vi "Cleanup.vi"(8 "error in (no error)":errorcluster, 11 "HAL Editor in":refnum<class "HAL Editor.lvclass">) -> (0 "error out":errorcluster)   [LabVIEW 2012, in "HAL Config.lvlib" / "HAL Editor.lvclass"]
uses:
  HAL Editor.lvclass
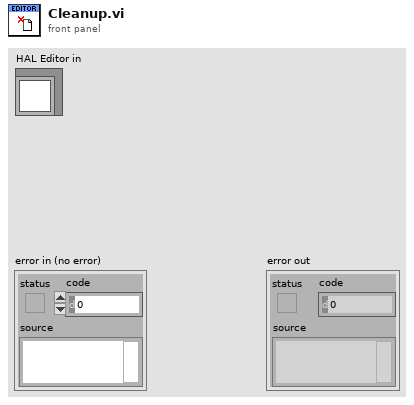
[diagram p1: front panel]
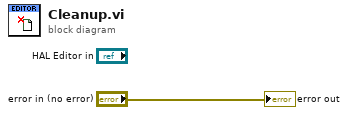
[diagram p0: block diagram]
diagram:
  "error out" <- "error in (no error)"
